vi "Accelration Control (by Throttle) V2.vi"(2 "acc":dbl, 3 "Hand break":bool, 4 "Yinput":dbl, 5 "Xinput":dbl) -> (0 "Youtput":dbl format="%.2f", 1 "Xoutput":dbl format="%.2f")   [LabVIEW 2012]
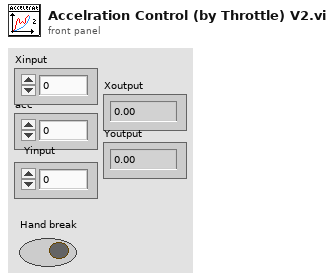
[diagram p1: front panel]
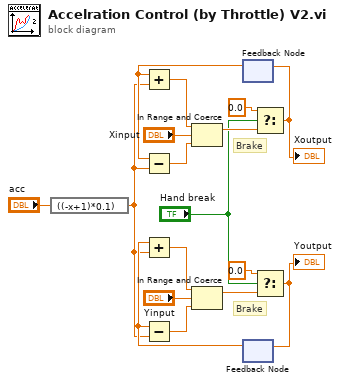
[diagram p0: block diagram]
diagram:
  # "Brake"
  # "Brake"
  n1 = expression code="((-x+1)*0.1)"("acc") -> (w2:dbl)
  n2 = feedback #1() -> (w15:dbl)  [unwired: 1 in]
  n3 = Add(x=w15, y=w2) -> (x+y=w16:dbl)
  n4 = Subtract(x=w15, y=w2) -> (x-y=w17:dbl)
  n5 = In Range and Coerce(upper limit=w16, x="Xinput", lower limit=w17) -> (coerced(x)=w12:dbl)  [unwired: 1 out]
  n6 = feedback #2() -> (w5:dbl)  [unwired: 1 in]
  n7 = Add(x=w5, y=w2) -> (x+y=w4:dbl)
  n8 = Subtract(x=w5, y=w2) -> (x-y=w3:dbl)
  n9 = In Range and Coerce(upper limit=w4, x="Yinput", lower limit=w3) -> (coerced(x)=w7:dbl)  [unwired: 1 out]
  n10 = Select(t=0.0, s="Hand break", f=w12) -> (s? t:f=w10:dbl)
  "Xoutput" <- w10
  n11 = feedback-in #1(w10) -> ()
  n12 = Select(t=0.0, s="Hand break", f=w7) -> (s? t:f=w9:dbl)
  "Youtput" <- w9
  n13 = feedback-in #2(w9) -> ()
